vi "algoritmo_7.vi"() -> ()   [LabVIEW 2024]
uses:
  <vilib>/Platform/TimedLoop/XDataNode/timing_clust.ctl
  <vilib>/Platform/TimedLoop/XDataNode/nitl_modes.ctl
  <vilib>/Platform/TimedLoop/XDataNode/wakeup.ctl
  <vilib>/MakerHub/LINX/Public/Peripherals/PWM/PWM Set Duty Cycle 1 Chan.vi
  <vilib>/MakerHub/LINX/Public/Utilities/Open Serial.vi
  <vilib>/MakerHub/LINX/Public/Peripherals/PWM/PWM Set Duty Cycle N Chans.vi
  <vilib>/platform/TimedLoop/XDataNode/XDataNode.xnode
  <vilib>/Platform/TimedLoop/XDataNode/XDNodeRunTimeDep.lvlib
  <vilib>/MakerHub/LINX/LMH-LINX.lvlib
  <vilib>/MakerHub/LINX/Public/Sensors/Distance/Ultrasonic/Ultrasonic.lvlib
  <vilib>/Analysis/NI_AALPro.lvlib
panel:
  out "m3":dbl
  out "m2":dbl
  out "m1":dbl
  out "UK":dbl
  out "Normal":dbl
  out "integral":dbl
  out "poli":dbl
  out "pb":dbl
  out "pa":dbl
  in  "pb":dbl(slide) scale=0.0..1.0
  in  "poli":dbl(slide) scale=0.0..1.0 scale format="%#_7g"
  in  "pol":dbl(slide) scale=-1.0..1.0 scale format="%#_7g"
  out "xk":dbl[](array[numeric])
  out "error":dbl
  in  "modo1":dbl(slide) scale=41.0..-41.0 scale format="%#_7g"
  in  "modo":dbl
  out "2-D Array of Complex":cdb[][](array[numeric])
  out "PWM":dbl format="%0.2f"
  out "estado":dbl
  out "MINUTOS":dbl format="%#_2g"
  out "y_estimada":dbl
  out "error de estimacion":dbl
  out "TETA":cdb[](array[numeric])
  out "Waveform Chart":T1(graph)
  in  "stop":bool
  in  "Serial Port":refnum<visa-resource-name>="N/A"
  out "Error Out":errorcluster
  in  "Referencia":dbl(slide) scale=40.0..5.0 scale format="%#_7g"
  out "Y_Real":fxp<+/-,64,32>
  # "1 PARA ESTIMAR"
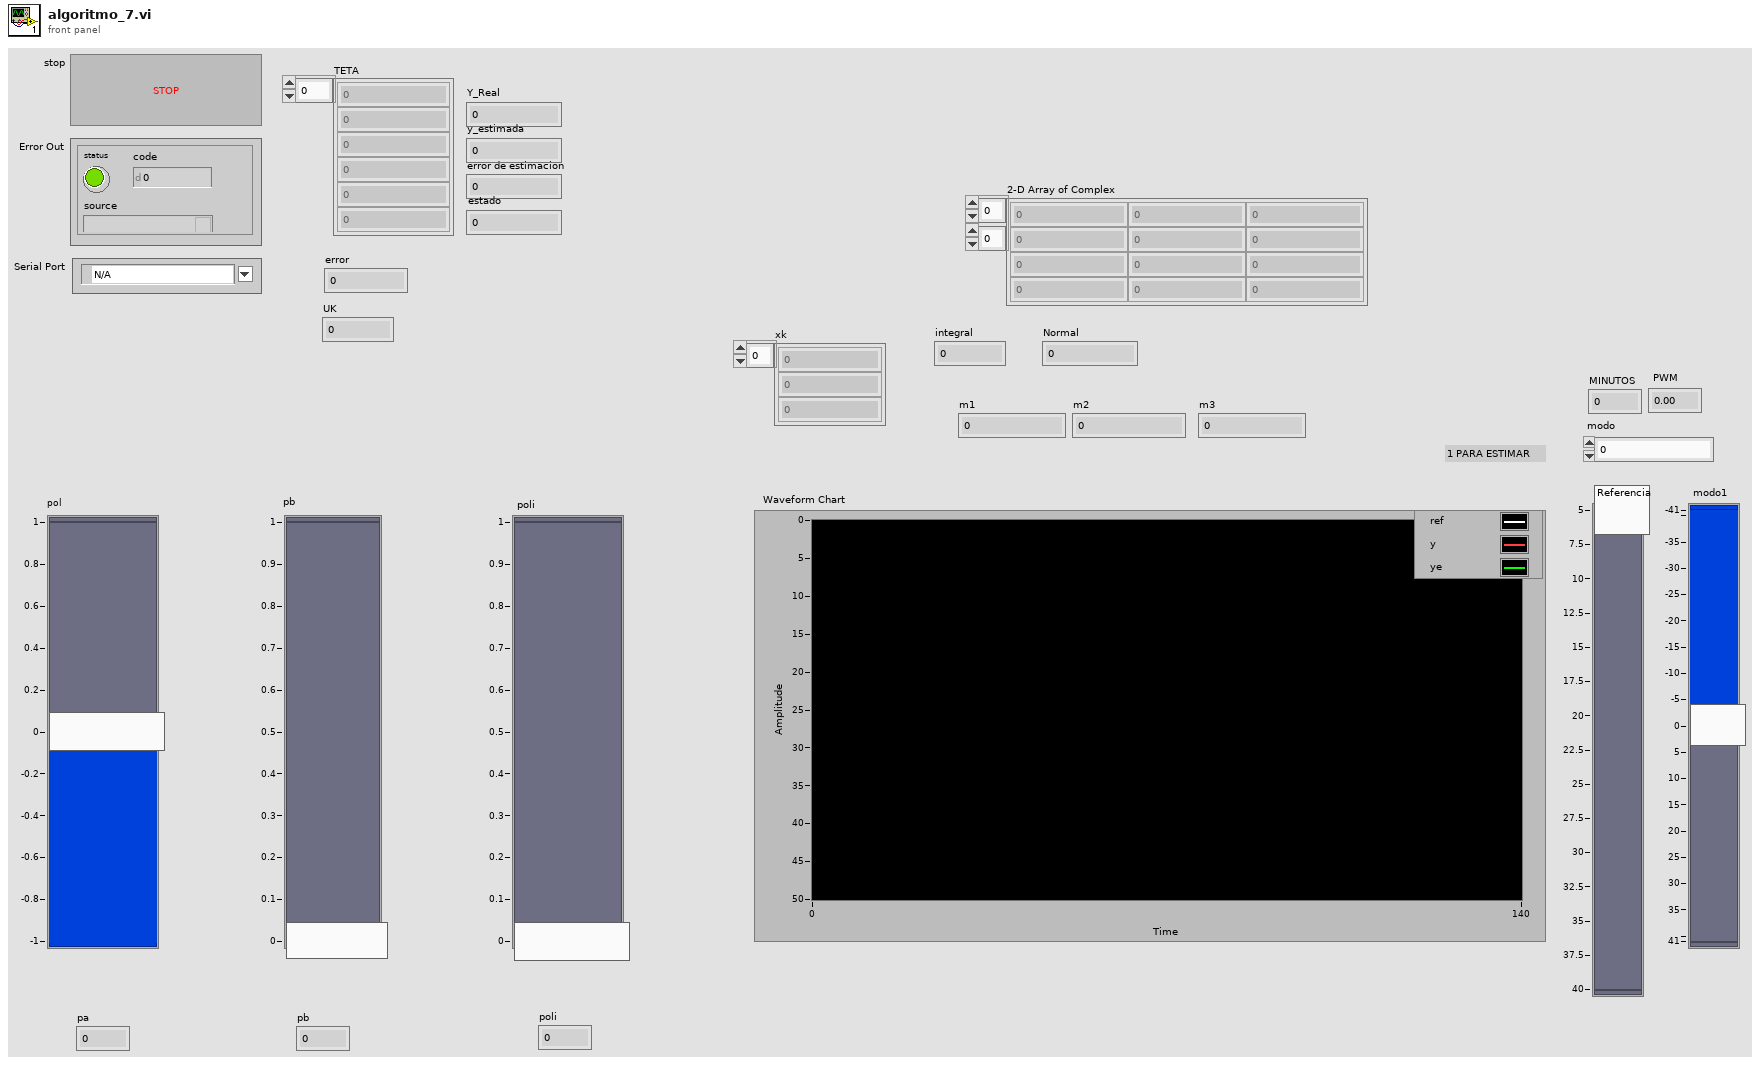
[diagram p1: front panel]
types:
  T1 = cluster{"Centimeters":dbl, "Referencia":dbl, dbl}
  T2 = typedef "LMH-LINX.lvlib/LINX Ref.ctl" = cluster{"IO":T3, "Interface":T4, "LINX Device Config":T5}
  T3 = typedef "LMH-LINX.lvlib/Platform.ctl" = enum16{"Remote", "Local"}
  T4 = typedef "LMH-LINX.lvlib/Interface.ctl" = enum16{"Serial", "TCP"}
  T5 = typedef "LMH-LINX.lvlib/Device.lvlib/LINX Device Config.ctl" = cluster{"Interface":T4, "COM Port":refnum<visa-resource-name>, "TCP Configuration":T6, "Device Family":u8, "Device ID":u8, "Device Name":string, "TCP Ref":refnum<k5>, "Channels":T7}
  T6 = typedef "LMH-LINX.lvlib/Device.lvlib/TCP Config.ctl" = cluster{"IP Address":string, "Port":u16}
  T7 = typedef "LMH-LINX.lvlib/Channels.ctl" = cluster{"DI":u8[], "DO":u8[], "AI":u8[], "AO":u8[], "PWM":u8[], "QE":u8[], "UART":u8[], "I2C 2":u8[], "SPI":u8[], "CAN":u8[], "Servo":u8[], "AI Ref (V)":dbl, "AI Resolution (Bits)":u8, "AO Ref (V)":dbl, "AO Resolution (Bits)":u8}
  T8 = typedef "XDNodeRunTimeDep.lvlib/timing_clust.ctl" = cluster{"Expected End [f-1]":u64, "Actual End [f-1]":u64, "Finished Late? [f-1]":bool, "Expected End [i-1]":u64, "Actual End [i-1]":u64, "Finished Late? [i-1]":bool, "Expected Start [i]":u64, "Actual Start [i]":u64, "Expected Start [f]":u64, "Actual Start [f]":u64, "Source Name":string, "Structure Name":string, "Period":i64, "Deadline":i64, "Offset":i64, "Start":i64, "Priority":i32, "Timeout":i32, "Mode":T9, "Wakeup Reason":T10, "Error":errorcluster, "Source Type":string, "Secondary Source Type":string, "Global End Time":u64, "Global Start Time":u64, "Frame Duration":u64, "Iteration Duration":u64, "Assigned CPU":i32, "I/O Scan Engine Mode":u32}
  T9 = typedef "XDNodeRunTimeDep.lvlib/nitl_modes.ctl" = enum32{"No Change", "Process missed periods, maintain original phase", "Discard missed periods, maintain original phase", "Process missed periods, ignore original phase", "Discard missed periods, ignore original phase"}
  T10 = typedef "XDNodeRunTimeDep.lvlib/wakeup.ctl" = enum32{"Normal", "Aborted", "Asynchronous wakeup", "Timing source error", "Timed loop error", "Timeout"}
  T11 = cluster{"Referencia":dbl, "Centimeters":dbl, dbl}
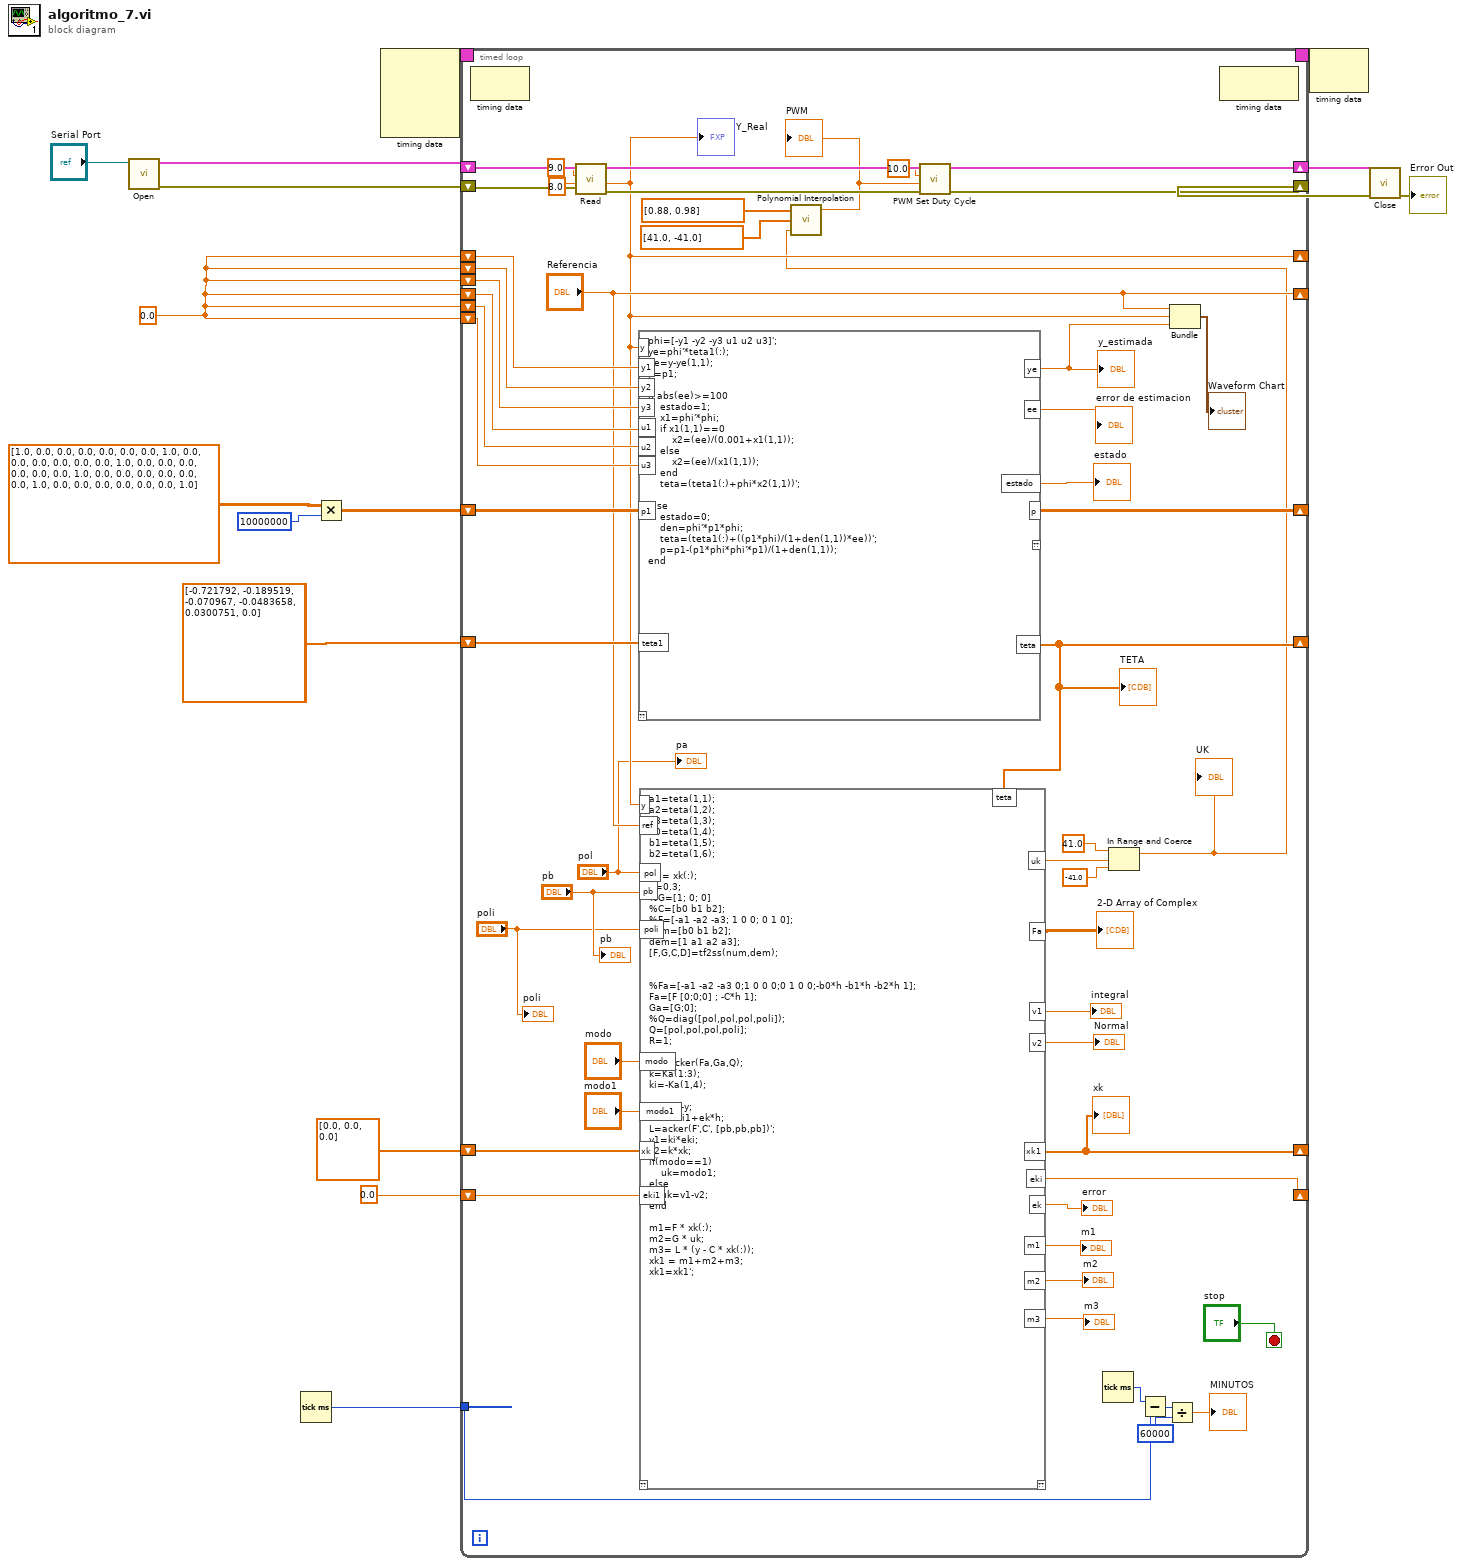
[diagram p0: block diagram]
diagram:
  (unwired) dbl[] [-1.03785, -0.0524271, 0.00439525, 0.0241947, 0.0113604, 0.0168977]
  w7 = 0.0
  n1 = call-poly <vilib>:"Open.vi"("Serial Port"="Serial Port") -> ("Error Out"=w12:errorcluster, "LINX Resource"=w14:T2)  [unwired: 8 in, 1 out]
  n2 = Tick Count (ms)() -> (millisecond timer value=w3:u32)
  n3 = Multiply(x=dbl[][] [[1.0, 0.0, 0.0, 0.0, 0.0, 0.0], [0.0, 1.0, 0.0, 0.0, 0.0, 0.0], [0.0, 0.0, 1.0, 0.0, 0.0, 0.0], [0.0, 0.0, 0.0, 1.0, 0.0, 0.0], [0.0, 0.0, 0.0, 0.0, 1.0, 0.0], [0.0, 0.0, 0.0, 0.0, 0.0, 1.0]], y=10000000) -> (x*y=w4:dbl[][])
  n4 = node-c288() -> (w16:T8)  [unwired: 4 in]
  n5 = timed-loop {
    timing: w16 -> [_]
    timing-out: [_] -> w15
    shift-right: [w59] -> w13
    shift-left: w14 -> [w70]
    shift-right: [w64] -> w11
    shift-left: w12 -> [w69]
    shift-right: [w39] -> _
    shift-left: dbl[] [-0.721792, -0.189519, -0.070967, -0.0483658, 0.0300751, 0.0] -> [w58]
    shift-right: [w35] -> _
    shift-left: w7 -> [w56]
    shift-right: ["Referencia"] -> _
    shift-left: w7 -> [w57]
    shift-left: w7 -> [w55]
    shift-left: w7 -> [w54]
    shift-left: w7 -> [w53]
    shift-left: w7 -> [w52]
    shift-right: [w49] -> _
    shift-left: w4 -> [w50]
    tunnel: w3 -> [w45]
    shift-right: [w25] -> _
    shift-left: dbl[] [0.0, 0.0, 0.0] -> [w37]
    shift-right: [w33] -> _
    shift-left: 0.0 -> [w34]
    stop <- "stop" stop-if-true
    n6 = node-c288() -> ()  [unwired: 1 in, 1 out]
    n7 = call <vilib>:"Read.vi"("Error In"=w69, "DO Channel"=8.0, "DI Channel"=9.0, "LINX Resource"=w70) -> ("Error Out"=w65:errorcluster, "Centimeters"=w35:dbl, "LINX Resource"=w66:T2)  [unwired: 4 in, 1 out]
    "Y_Real" <- w35
    n8 = script code="phi=[-y1 -y2 -y3 u1 u2 u3]';\nye=phi'*teta1(:);\nee=y-ye(1,1);\np=p1;\n\nif abs(ee)>=100\n    estado=1;\n    x1=phi'*phi;\n    if x1(1,1)==0\n        x2=(ee)/(0.001+x1(1,1));\n    else\n        x2=(ee)/(x1(1,1));\n    end\n    teta=(teta1(:)+phi*x2(1,1))';\n\nelse\n    estado=0;\n    den=phi'*p1*phi;\n    teta=(teta1(:)+((p1*phi)/(1+den(1,1))*ee))';\n    p=p1-(p1*phi*phi'*p1)/(1+den(1,1));\nend"("teta1"=w58, "y1"=w56, "y2"=w55, "y3"=w54, "u1"=w57, "u2"=w53, "u3"=w52, "y"=w35, "p1"=w50) -> ("teta"=w39:dbl[], "p"=w49:dbl[][], "ye"=w48:dbl, "ee"=→"error de estimacion":dbl, "estado"=→"estado":dbl)  [unwired: 1 in, 1 out]
    "TETA" <- w39
    "y_estimada" <- w48
    n9 = script code="a1=teta(1,1);\na2=teta(1,2);\na3=teta(1,3);\nb0=teta(1,4);\nb1=teta(1,5);\nb2=teta(1,6);\n\nxk = xk(:);\nh=0.3;\n%G=[1; 0; 0]\n%C=[b0 b1 b2];\n%F=[-a1 -a2 -a3; 1 0 0; 0 1 0];\nnum=[b0 b1 b2];\ndem=[1 a1 a2 a3];\n[F,G,C,D]=tf2ss(num,dem); \n\n\n%Fa=[-a1 -a2 -a3 0;1 0 0 0;0 1 0 0;-b0*h -b1*h -b2*h 1];\nFa=[F [0;0;0] ; -C*h 1];\nGa=[G;0];\n%Q=diag([pol,pol,pol,poli]);\nQ=[pol,pol,pol,poli];\nR=1;\n\nKa=acker(Fa,Ga,Q);\nk=Ka(1:3);\nki=-Ka(1,4);\n\nek=ref-y;\neki=eki1+ek*h;\nL=acker(F',C', [pb,pb,pb])';\nv1=ki*eki;\nv2=k*xk;\nif(modo==1)\n    uk=modo1;\nelse    \n    uk=v1-v2;\nend\n\nm1=F * xk(:);\nm2=G * uk;\nm3= L * (y - C * xk(:));\nxk1 = m1+m2+m3;\nxk1=xk1';"("teta"=w39, "pol"="pol", "poli"="poli", "ref"="Referencia", "y"=w35, "xk"=w37, "eki1"=w34, "modo"="modo", "modo1"="modo1", "pb"="pb") -> ("Fa"=→"2-D Array of Complex":cdb[][], "xk1"=w25:dbl[], "eki"=w33:dbl, "uk"=w28:dbl, "ek"=→"error":dbl, "v1"=→"integral":dbl, "v2"=→"Normal":dbl, "m1"=→"m1":dbl, "m2"=→"m2":dbl, "m3"=→"m3":dbl)  [unwired: 1 in, 1 out]
    "xk" <- w25
    n10 = Tick Count (ms)() -> (millisecond timer value=w46:u32)
    n11 = In Range and Coerce(upper limit=41.0, x=w28, lower limit=-41.0) -> (coerced(x)=w27:dbl)  [unwired: 1 out]
    "UK" <- w27
    n12 = call <vilib>:"Polynomial Interpolation.vi"("x value"=w27, "X"=dbl[] [41.0, -41.0], "Y"=dbl[] [0.88, 0.98]) -> ("interpolation value"=w40:dbl)  [unwired: 2 out]
    "PWM" <- w40
    n13 = call-poly <vilib>:"PWM Set Duty Cycle.vi"("Error In"=w65, "Duty Cycle (0-1)"=w40, "PWM Channel"=10.0, "LINX Resource"=w66) -> ("Error Out"=w64:errorcluster, "LINX Resource"=w59:T2)  [unwired: 6 in]
    n14 = Subtract(x=w46, y=w45) -> (x-y=w43:u32)
    n15 = Divide(x=w43, y=u32 60000) -> (x/y=→"MINUTOS":dbl)
    n16 = Bundle("Referencia"="Referencia", "Centimeters"=w35, w48) -> (→"Waveform Chart":T11)  [unwired: 1 in]
    n17 = node-c288() -> ()  [unwired: 1 in, 1 out]
    "poli" <- "poli"
    "pb" <- "pb"
    "pa" <- "pol"
  }
  n18 = node-c288(w15) -> ()  [unwired: 1 out]
  n19 = call <vilib>:"Close.vi"("Error In"=w11, "LINX Resource"=w13) -> ("Error Out"=→"Error Out":errorcluster)  [unwired: 9 in]
